vi "Sine Wave Chart [While loop].vi"() -> ()   [LabVIEW 2017]
panel:
  in  "Stop":bool
  out "Waveform Chart":dbl(graph)
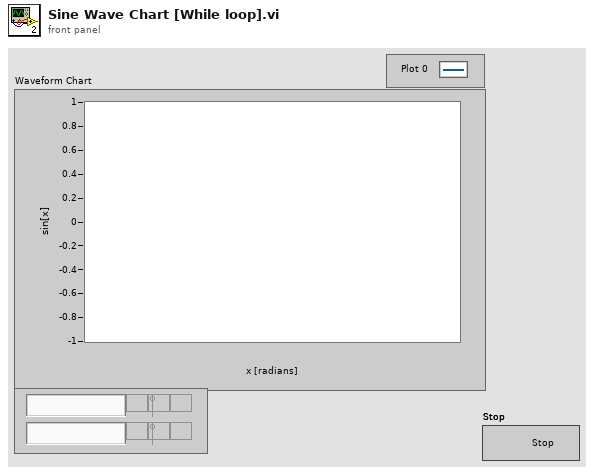
[diagram p1: front panel]
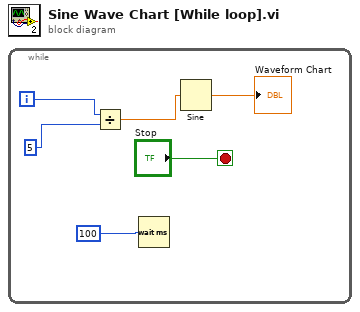
[diagram p0: block diagram]
diagram:
  n1 = while {
    i -> [w2]
    stop <- "Stop" stop-if-true
    n2 = Divide(x=w2, y=5) -> (x/y=w1:dbl)
    n3 = Wait (ms)(milliseconds to wait=u32 100) -> ()  [unwired: 1 out]
    n4 = Sine(x=w1) -> (sin(x)=→"Waveform Chart":dbl)
  }
